vi "Kicker_Control.vi"() -> ()   [LabVIEW 2017]
doc: "The myRIO Project template acquires acceleration data from the onboard accelerometer and displays the changes of acceleration values in a waveform chart."
panel:
  out "Process complete":bool
  in  "Release Mag":bool=TRUE
  in  "Desired Theta Angle":dbl(knob) step=0.9 scale=-90.0..90.0
  in  "Continue":bool
  out "Error Out":errorcluster
  in  "Error In":errorcluster
  in  "Stop":bool
  in  "START":bool
  in  "Required Pos":dbl(slide)=20.0 step=1.0 scale=0.0..100.0 scale format="%#_3g%%"
  # "Kicker Plate Collection"
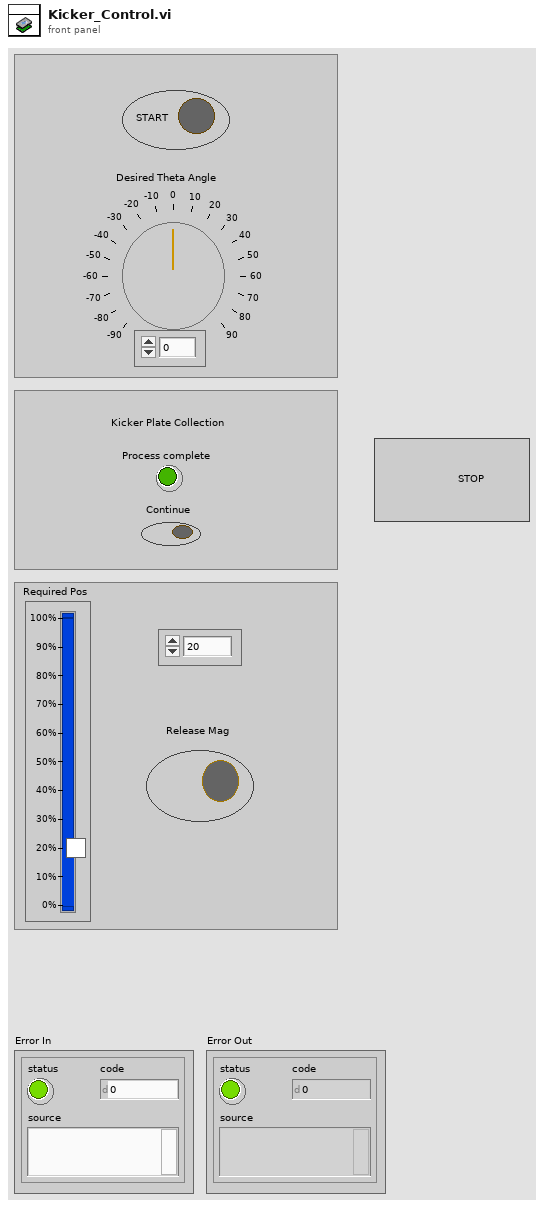
[diagram p1: front panel]
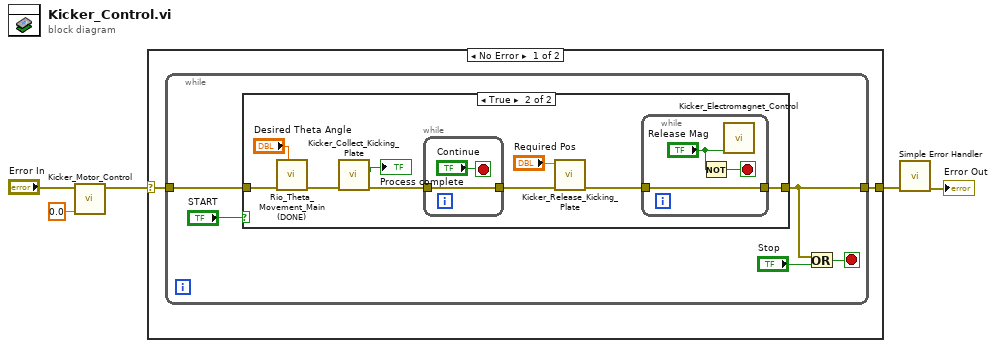
[diagram p0: block diagram]
diagram:
  n1 = call "Kicker_Motor_Control.vi"("Duty Cycle"=0.0, "error in"="Error In") -> ("error out"=w3:errorcluster)  [unwired: 9 in]
  n2 = case shown="No Error" w3 {
    selector: w3 -> [w6 w28]
    tunnel: [w7 w28] -> w5
    frame No Error {
      n3 = while {
        tunnel: [w9] -> w7
        tunnel: w6 -> [w8]
        stop <- w10 stop-if-true
        n4 = case shown="True" "START" {
          tunnel: [w13 w15] -> w9
          tunnel: w8 -> [w13 w19]
          frame False {
          }
          frame True {
            n5 = call "Rio_Theta_Movement_Main (DONE).vi"("Desired Position"="Desired Theta Angle", "Error In"=w19) -> ("error out"=w18:errorcluster)  [unwired: 9 in]
            n6 = call "Kicker_Collect_Kicking_Plate.vi"("error in"=w18) -> ("error out"=w21:errorcluster, "Boolean"=→"Process complete":bool)  [unwired: 8 in, 1 out]
            n7 = while {
              tunnel: w21 -> [w26]
              tunnel: [w26] -> w20
              stop <- "Continue" stop-if-true
            }
            n8 = call "Kicker_Release_Kicking_Plate.vi"("error in"=w20, "Required Pos"="Required Pos") -> ("error out"=w16:errorcluster)  [unwired: 8 in, 1 out]
            n9 = while {
              tunnel: w16 -> [w25]
              tunnel: [w25] -> w15
              stop <- w23 stop-if-true
              n10 = Not(x="Release Mag") -> (.not. x?=w23:bool)
              n11 = call "Kicker_Electromagnet_Control.vi"("Mag Enable"="Release Mag") -> ()  [unwired: 10 in, 1 out]
            }
          }
        }
        n12 = Or(x=w9, y="Stop") -> (x .or. y?=w10:bool)
      }
    }
    frame Error {
    }
  }
  n13 = call <vilib>:"Simple Error Handler.vi"("error in (no error)"=w5) -> ("error out"=→"Error Out":errorcluster)  [unwired: 4 in, 4 out]
